vi "Command Parameters FG.vi"(7 "Action":T1, 8 "error in (no error)":errorcluster, 10 "Command Parameters":T3={"Command"="", "Linked Channels"=[], "Pad"=FALSE, "Length"=25, "Pad Value"=0}, 11 "Item Ref in":T2 format="%.0x") -> (0 "error out":errorcluster, 2 "Command Parameters":T3={"Command"="", "Linked Channels"=[], "Pad"=FALSE, "Length"=25, "Pad Value"=0}, 3 "Item Ref out":T2 format="%.0x")   [LabVIEW 2020, in "Instrument Addon Shared.lvlib"]
uses:
  Instrument Addon Shared.lvlib
  Command Parameters.ctl
  Linked Channel Cluster.ctl
  <vilib>/NI VeriStand/Custom Device API/Custom Device Item Ref.ctl
  FG Control.ctl
  Constants.vi
  <vilib>/NI VeriStand/Custom Device API/Get Item Property (String).vi
  <vilib>/NI VeriStand/Custom Device API/Get Item Property (String Array).vi
  <vilib>/NI VeriStand/Custom Device API/Get Item Property (Boolean).vi
  <vilib>/NI VeriStand/Custom Device API/Get Item Property (U32).vi
  <vilib>/NI VeriStand/Custom Device API/Set Item Property (String).vi
  <vilib>/NI VeriStand/Custom Device API/Set Item Property (String Array).vi
  <vilib>/NI VeriStand/Custom Device API/Set Item Property (Boolean).vi
  <vilib>/NI VeriStand/Custom Device API/Set Item Property (U32).vi
  <vilib>/NI VeriStand/Custom Device API/Custom Device API.lvlib
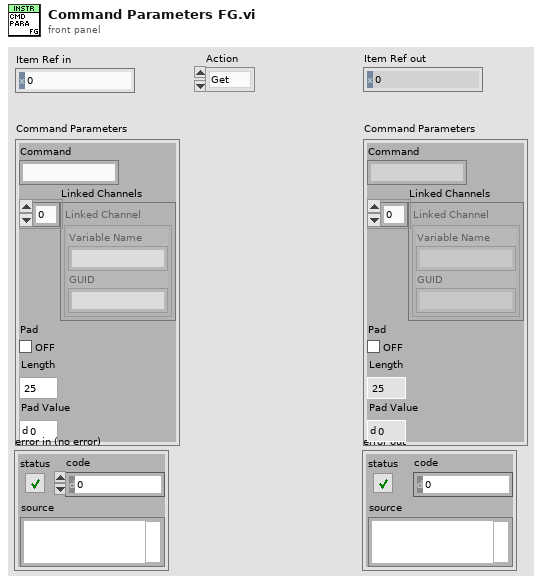
[diagram p1: front panel]
types:
  T1 = typedef "Instrument Addon Shared.lvlib/FG Control.ctl" = enum16{"Get", "Set"}
  T2 = typedef "Custom Device API.lvlib/Custom Device Item Ref.ctl" = u64
  T3 = typedef "Instrument Addon Shared.lvlib/Command Parameters.ctl" = cluster{"Command":string, "Linked Channels":T4[], "Pad":bool, "Length":u32, "Pad Value":u8}
  T4 = typedef "Instrument Addon Shared.lvlib/Linked Channel Cluster.ctl" = cluster{"Variable Name":string, "GUID":string}
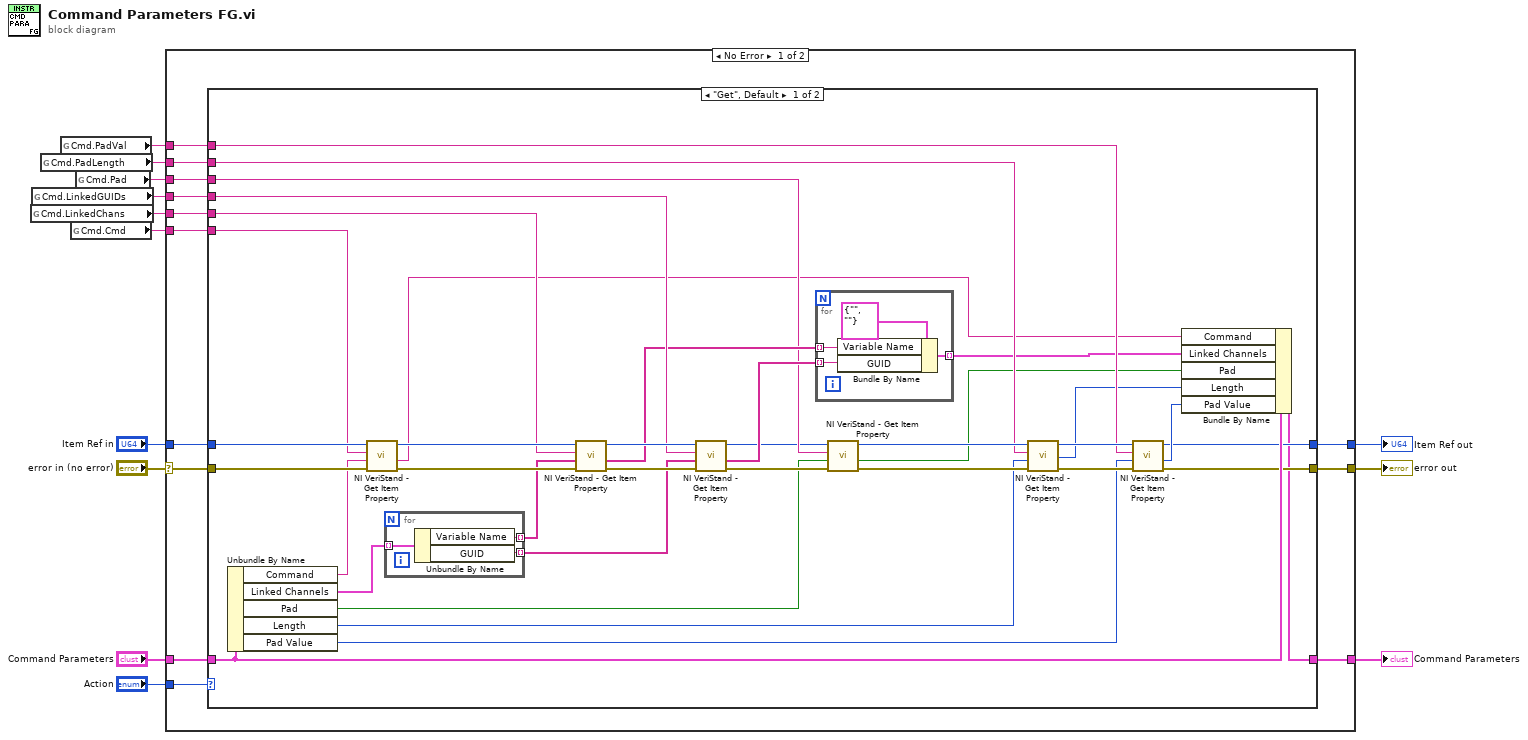
[diagram p0: block diagram]
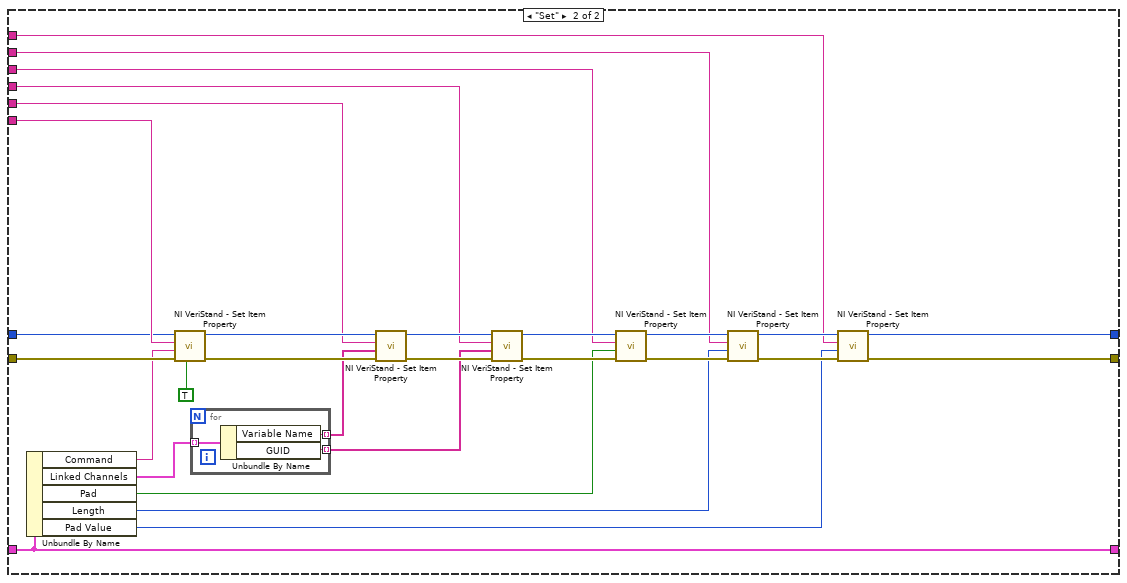
[diagram p2: hidden frame]
diagram:
  n1 = global read "Constants.vi" "Cmd.LinkedChans"() -> (w5:string)
  n2 = global read "Constants.vi" "Cmd.LinkedGUIDs"() -> (w4:string)
  n3 = global read "Constants.vi" "Cmd.PadLength"() -> (w2:string)
  n4 = global read "Constants.vi" "Cmd.PadVal"() -> (w1:string)
  n5 = global read "Constants.vi" "Cmd.Cmd"() -> (w7:string)
  n6 = global read "Constants.vi" "Cmd.Pad"() -> (w3:string)
  n7 = case shown="No Error" "error in (no error)" {
    selector: "error in (no error)" -> [w21 w104]
    tunnel: w7 -> [w26 _]
    tunnel: [w25 w102] -> w11
    tunnel: "Item Ref in" -> [w24 w102]
    tunnel: "Command Parameters" -> [w23 w103]
    tunnel: [w22 w104] -> w10
    tunnel: [w20 w103] -> w6
    tunnel: "Action" -> [w19 _]
    tunnel: w5 -> [w18 _]
    tunnel: w4 -> [w17 _]
    tunnel: w3 -> [w16 _]
    tunnel: w2 -> [w15 _]
    tunnel: w1 -> [w14 _]
    frame No Error {
      n8 = case shown="\"Get\", Default" w19 {
        tunnel: w26 -> [w60 w98]
        tunnel: [w29 w70] -> w25
        tunnel: w24 -> [w61 w97]
        tunnel: w23 -> [w35 w95]
        tunnel: [w30 w71] -> w22
        tunnel: w21 -> [w62 w96]
        tunnel: [w28 w95] -> w20
        tunnel: w18 -> [w48 w81]
        tunnel: w17 -> [w47 w80]
        tunnel: w16 -> [w43 w76]
        tunnel: w15 -> [w37 w75]
        tunnel: w14 -> [w36 w72]
        frame "Get", Default {
          n9 = Unbundle By Name(w35) -> ("Command"=w53:string, "Linked Channels"=w52:T4[], "Pad"=w44:bool, "Length"=w41:u32, "Pad Value"=w40:u8)
          n10 = call-poly <vilib>:"NI VeriStand - Get Item Property.vi"("error in (no error)"=w62, "Default Value"=w53, "Property Name"=w60, "Item Ref in"=w61) -> ("error out"=w59:errorcluster, "Value"=w27:string, "Item Ref out"=w58:T2)  [unwired: 4 in, 1 out]
          n11 = for {
            tunnel: w52 -> [w69] mode=indexing
            tunnel: [w68] -> w51 mode=indexing
            tunnel: [w67] -> w50 mode=indexing
            n12 = Unbundle By Name(w69) -> ("Variable Name"=w68:string, "GUID"=w67:string)
          }
          n13 = call-poly <vilib>:"NI VeriStand - Get Item Property.vi"("error in (no error)"=w59, "Default Value"=w51, "Property Name"=w48, "Item Ref in"=w58) -> ("error out"=w57:errorcluster, "Value"=w45:string[], "Item Ref out"=w49:T2)  [unwired: 4 in, 1 out]
          n14 = call-poly <vilib>:"NI VeriStand - Get Item Property.vi"("error in (no error)"=w57, "Default Value"=w50, "Property Name"=w47, "Item Ref in"=w49) -> ("error out"=w56:errorcluster, "Value"=w46:string[], "Item Ref out"=w42:T2)  [unwired: 4 in, 1 out]
          n15 = for {
            tunnel: w46 -> [w64] mode=indexing
            tunnel: w45 -> [w63] mode=indexing
            tunnel: [w65] -> w34 mode=indexing
            n16 = Bundle By Name(cluster=T4 {"Variable Name"="", "GUID"=""} ("Linked Channel"), "Variable Name"=w63, "GUID"=w64) -> (w65:T4)
          }
          n17 = call-poly <vilib>:"NI VeriStand - Get Item Property.vi"("error in (no error)"=w56, "Default Value"=w44, "Property Name"=w43, "Item Ref in"=w42) -> ("error out"=w55:errorcluster, "Value"=w33:bool, "Item Ref out"=w38:T2)  [unwired: 4 in, 1 out]
          n18 = call-poly <vilib>:"NI VeriStand - Get Item Property.vi"("error in (no error)"=w55, "Default Value"=w41, "Property Name"=w37, "Item Ref in"=w38) -> ("error out"=w54:errorcluster, "Value"=w32:u32, "Item Ref out"=w39:T2)  [unwired: 4 in, 1 out]
          n19 = call-poly <vilib>:"NI VeriStand - Get Item Property.vi"("error in (no error)"=w54, "Default Value"=w40, "Property Name"=w36, "Item Ref in"=w39) -> ("error out"=w30:errorcluster, "Value"=w31:u32, "Item Ref out"=w29:T2)  [unwired: 4 in, 1 out]
          n20 = Bundle By Name(cluster=w35, "Command"=w27, "Linked Channels"=w34, "Pad"=w33, "Length"=w32, "Pad Value"=w31) -> (w28:T3)
        }
        frame "Set" {
          n21 = Unbundle By Name(w95) -> ("Command"=w94:string, "Linked Channels"=w92:T4[], "Pad"=w77:bool, "Length"=w74:u32, "Pad Value"=w73:u8)
          n22 = call-poly <vilib>:"NI VeriStand - Set Item Property.vi"("Binary String (T)"=TRUE, "error in (no error)"=w96, "Value"=w94, "Property Name"=w98, "Item Ref in"=w97) -> ("error out"=w90:errorcluster, "Item Ref out"=w91:T2)  [unwired: 4 in, 1 out]
          n23 = for {
            tunnel: w92 -> [w101] mode=indexing
            tunnel: [w100] -> w78 mode=indexing
            tunnel: [w99] -> w79 mode=indexing
            n24 = Unbundle By Name(w101) -> ("Variable Name"=w100:string, "GUID"=w99:string)
          }
          n25 = call-poly <vilib>:"NI VeriStand - Set Item Property.vi"("error in (no error)"=w90, "Value"=w78, "Property Name"=w81, "Item Ref in"=w91) -> ("error out"=w89:errorcluster, "Item Ref out"=w82:T2)  [unwired: 5 in, 1 out]
          n26 = call-poly <vilib>:"NI VeriStand - Set Item Property.vi"("error in (no error)"=w89, "Value"=w79, "Property Name"=w80, "Item Ref in"=w82) -> ("error out"=w88:errorcluster, "Item Ref out"=w83:T2)  [unwired: 5 in, 1 out]
          n27 = call-poly <vilib>:"NI VeriStand - Set Item Property.vi"("error in (no error)"=w88, "Value"=w77, "Property Name"=w76, "Item Ref in"=w83) -> ("error out"=w87:errorcluster, "Item Ref out"=w84:T2)  [unwired: 5 in, 1 out]
          n28 = call-poly <vilib>:"NI VeriStand - Set Item Property.vi"("error in (no error)"=w87, "Value"=w74, "Property Name"=w75, "Item Ref in"=w84) -> ("error out"=w86:errorcluster, "Item Ref out"=w85:T2)  [unwired: 5 in, 1 out]
          n29 = call-poly <vilib>:"NI VeriStand - Set Item Property.vi"("error in (no error)"=w86, "Value"=w73, "Property Name"=w72, "Item Ref in"=w85) -> ("error out"=w71:errorcluster, "Item Ref out"=w70:T2)  [unwired: 5 in, 1 out]
        }
      }
    }
    frame Error {
    }
  }
  "error out" <- w10
  "Command Parameters" <- w6
  "Item Ref out" <- w11
